vi "VHM-sendVNASettings.vi"(8 "error in (no error)":errorcluster, 11 "VHM-VNA_Hardware_Manager in":refnum<class "VHM-VNA_Hardware_Manager.lvclass">) -> (0 "error out":errorcluster, 3 "VHM-VNA_Hardware_Manager out":refnum<class "VHM-VNA_Hardware_Manager.lvclass">)   [LabVIEW 2020, in "VHM-VNA_Hardware_Manager.lvlib" / "VHM-VNA_Hardware_Manager.lvclass"]
uses:
  VHM-VNA_Hardware_Manager.lvclass
  VHM-VNA_Hardware_Manager.lvclass/VHM-VNA_Hardware_Manager.ctl
  VHMI-VNA_Hardware_manager_Interface Messages/VHMI-recieveSettings Msg/VHMI-recieveSettings Msg.lvclass/VHMI-recieveSettings Msg.ctl
  <vilib>/ActorFramework/Message Enqueuer/Message Enqueuer.lvclass/Message Enqueuer.ctl
  <vilib>/ActorFramework/Message Enqueuer/Enqueue.vi
  VHMI-VNA_Hardware_manager_Interface Messages/VHMI-recieveSettings Msg/VHMI-recieveSettings Msg.lvclass
  C:/Program Files (x86)/National Instruments/LabVIEW 2020/vi.lib/ActorFramework/Message/Message.lvclass
  <vilib>/ActorFramework/Message Priority Queue/Priority Enqueue.vi
  classes/vna-drivers/liteVNA/VD-LV-LiteVNA.lvclass
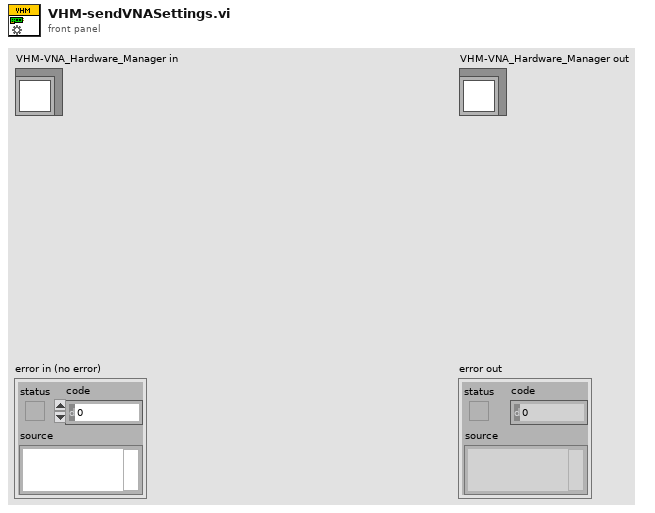
[diagram p1: front panel]
types:
  T1 = typedef "VD-LV-LiteVNA.lvclass/VD-settings_status.ctl" = cluster{"Start [Hz]":u64, "Span [Hz]":u64, "Stop [Mhz]":u64, "Number of points #":u16, "Sample Average #":u16}
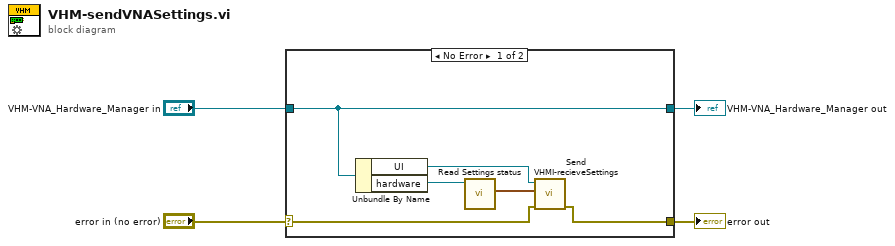
[diagram p0: block diagram]
diagram:
  n1 = case shown="No Error" "error in (no error)" {
    selector: "error in (no error)" -> [w6 w12]
    tunnel: [w5 w12] -> w3
    tunnel: [w10 w11] -> w1
    tunnel: "VHM-VNA_Hardware_Manager in" -> [w10 w11]
    frame No Error {
      n2 = Unbundle By Name(w10) -> ("UI"=w7:refnum<class "Message Enqueuer.lvclass">, "hardware"=w9:refnum<class "VD-LV-LiteVNA.lvclass">)
      n3 = call-dynamic "Read Settings status.vi"("VD-LV-LiteVNA in"=w9) -> ("Settings"=w8:T1)  [unwired: 8 in, 2 out]
      n4 = call "Send VHMI-recieveSettings.vi"("error in (no error)"=w6, "Settings"=w8, "Message Enqueuer"=w7) -> ("error out"=w5:errorcluster)  [unwired: 7 in, 1 out]
    }
    frame Error {
    }
  }
  "error out" <- w3
  "VHM-VNA_Hardware_Manager out" <- w1
